vi "Cube Manipulation Logic Core v2.vi"(6 "Auto Control":bool, 8 "Manual Intake Control":dbl, 9 "Manual Lift Control":dbl, 10 "Cube Manipulation Manual Controls":T1, 11 "Cube Manipulation Button Controls":T4) -> (3 "output cluster":T2={"Control Mode"=1, "Carrage Output"=0.0, "Intake Output"=0.0, "Intake Short"=FALSE, "Intake Long"=FALSE, "Lift Output"=0.0, "Lift Output L"=0.0, "Lift Output R"=0.0} {"Control Mode" items=["PercentOutput"=0, "Position"=1, "Velocity"=2, "Current"=3, "Follower"=5, "MotionProfile"=6, "MotionMagic"=7, "MotionMagicArc"=8, "MotionProfileArc"=10, "Disabled"=15]}, 5 "Sequence Done":bool, 7 "Position Reached":bool)   [LabVIEW 2017]
uses:
  Cube Manipulation Controls.ctl
  Cube Manipulation Outputs.ctl
  <vilib>/Rock Robotics/WPI/ThirdParty/Phoenix-LabVIEW/Motor Controller/Controls/CTRE_Phoenix_MotorControl_ControlMode.ctl
  Cube Manipulation Manual Controls.ctl
  Robot Global Data.vi
panel:
  in  "Case 0 Short Hold":bool
  in  "Adjust Grip Sequence":dbl
  in  "Solinoid Buffer for Positions":dbl=5000.0 format="%#_13g"
  in  "Exchange Sequence":dbl
  in  "Buffer Zone":dbl=3500.0
  in  "Command":dbl
  in  "Sequence Position":dbl
  # "Moved Wheel \nSpeed to Global"
  # "Off= Retracted\nOn= Extended"
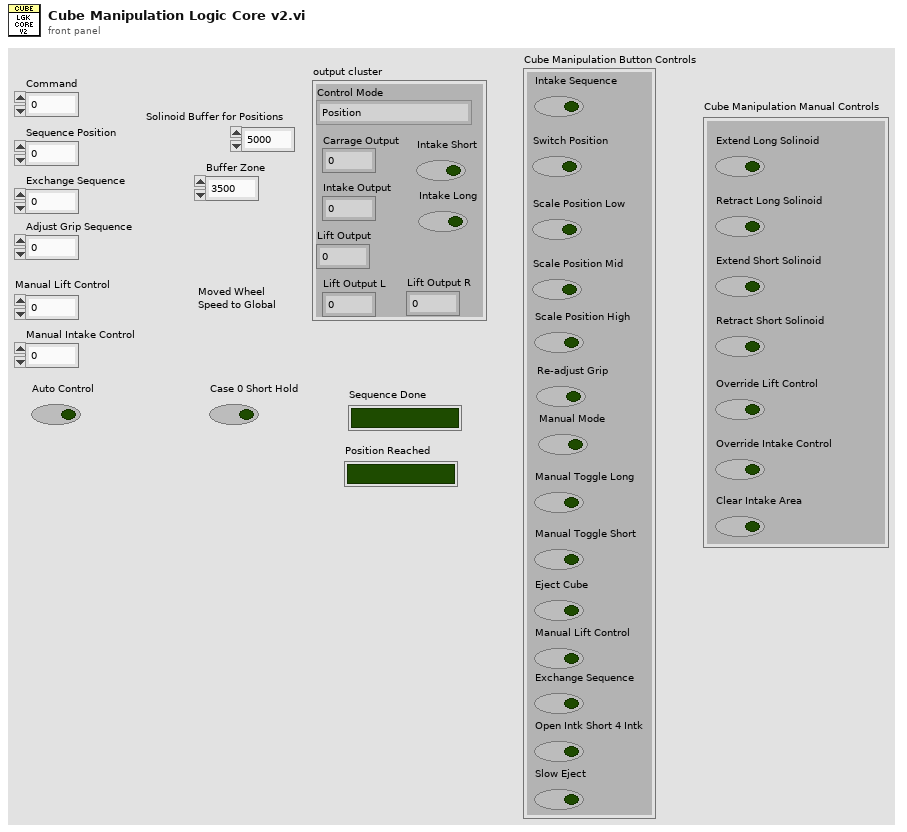
[diagram p1: front panel]
types:
  T1 = typedef "Cube Manipulation Manual Controls.ctl" = cluster{"Extend Long Solinoid":bool, "Retract Long Solinoid":bool, "Extend Short Solinoid":bool, "Retract Short Solinoid":bool, "Override Lift Control":bool, "Override Intake Control":bool, "Clear Intake Area":bool}
  T2 = typedef "Cube Manipulation Outputs.ctl" = cluster{"Control Mode":T3, "Carrage Output":dbl, "Intake Output":dbl, "Intake Short":bool, "Intake Long":bool, "Lift Output":dbl, "Lift Output L":dbl, "Lift Output R":dbl}
  T3 = typedef "CTRE_Phoenix_MotorControl_ControlMode.ctl" = u16
  T4 = typedef "Cube Manipulation Controls.ctl" = cluster{"Intake Sequence":bool, "Switch Position":bool, "Scale Position Low":bool, "Scale Position Mid":bool, "Scale Position High":bool, "Re-adjust Grip":bool, "Manual Mode":bool, "Manual Toggle Long":bool, "Manual Toggle Short":bool, "Eject Cube":bool, "Manual Lift Control":bool, "Exchange Sequence":bool, "Open Intk Short 4 Intk":bool, "Slow Eject":bool}
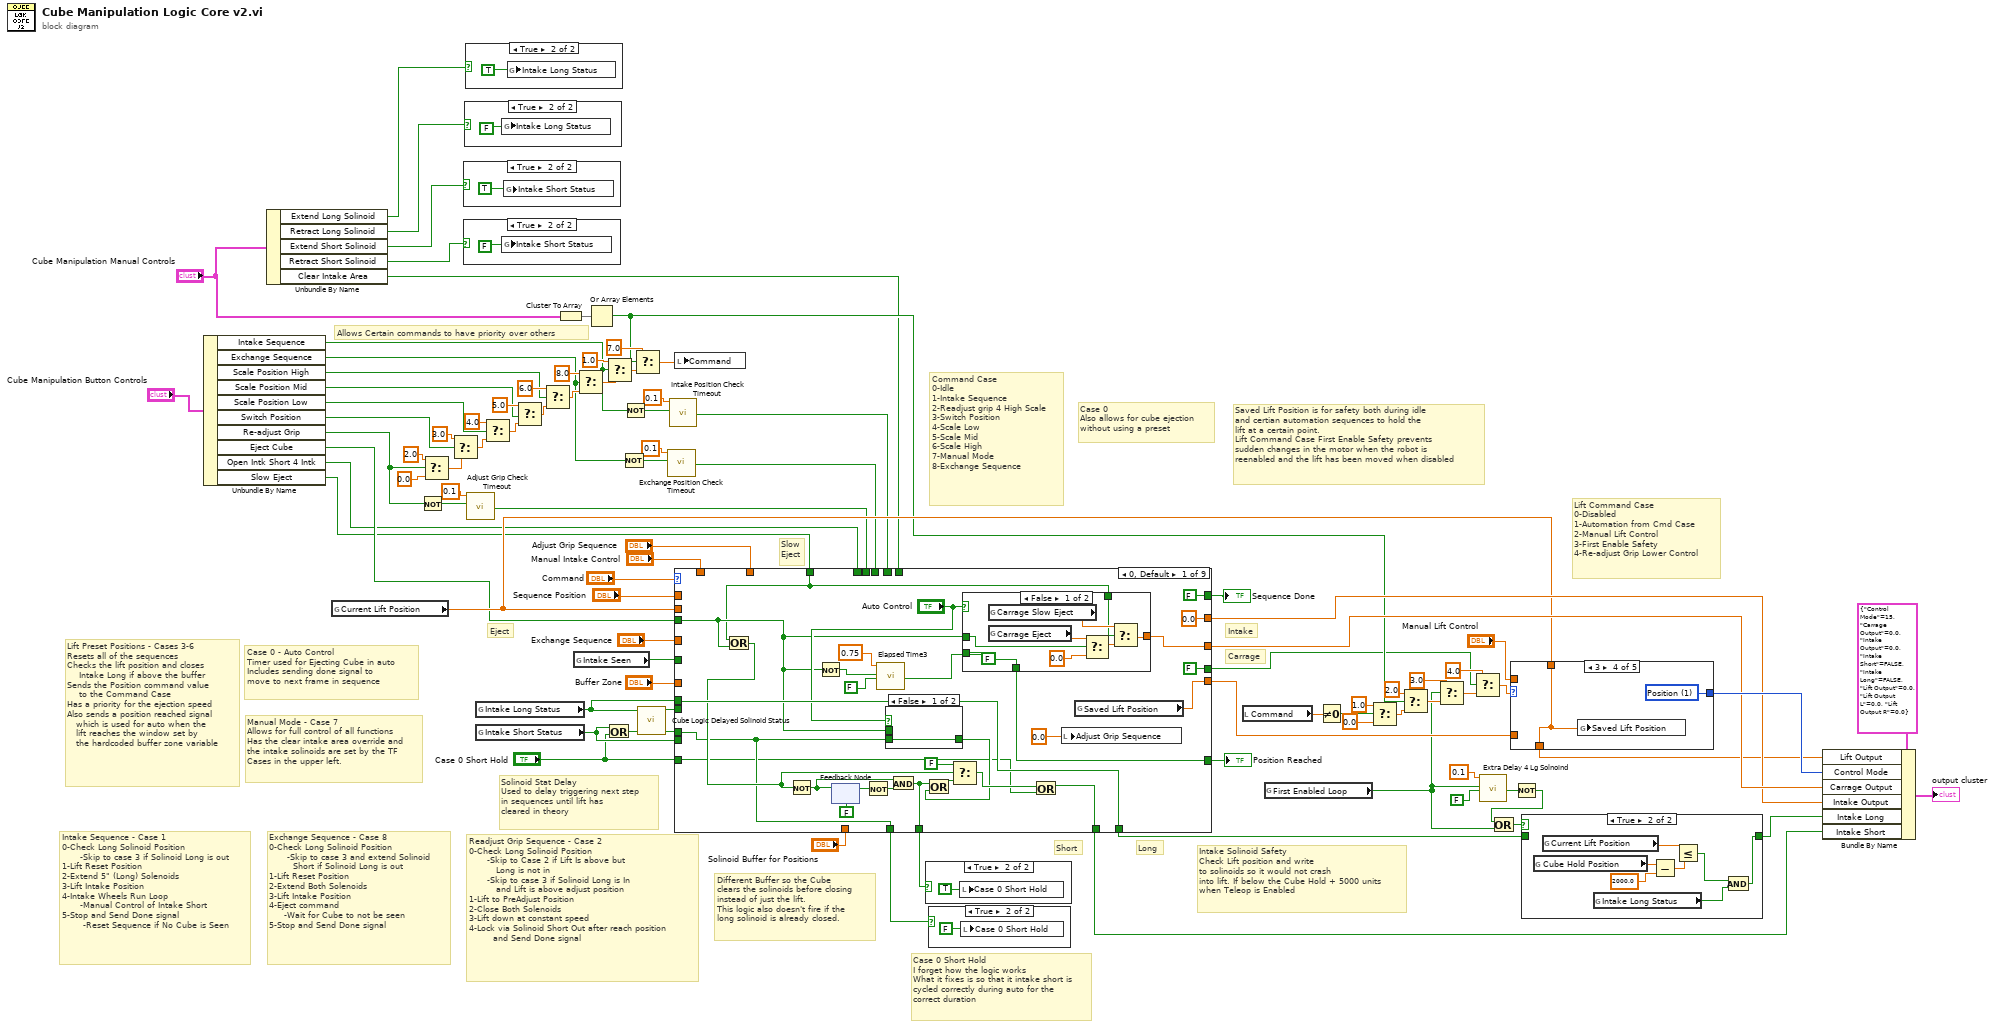
[diagram p0: block diagram]
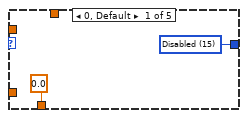
[diagram p9: hidden frame]
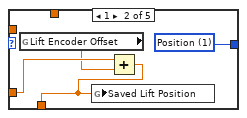
[diagram p10: hidden frame]
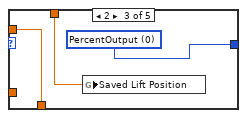
[diagram p11: hidden frame]
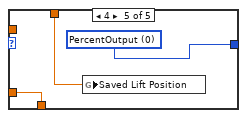
[diagram p12: hidden frame]
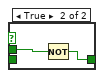
[diagram p13: hidden frame]
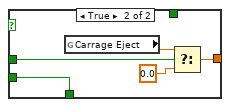
[diagram p14: hidden frame]
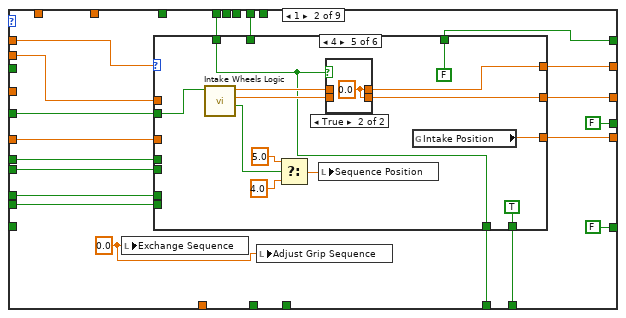
[diagram p15: hidden frame]
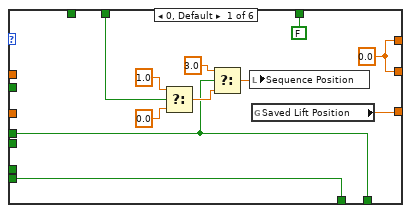
[diagram p16: hidden frame]
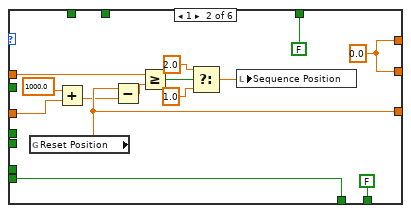
[diagram p17: hidden frame]
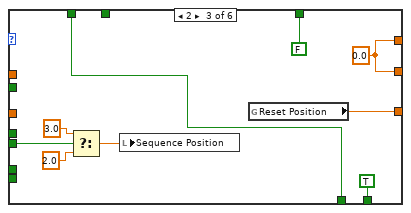
[diagram p18: hidden frame]
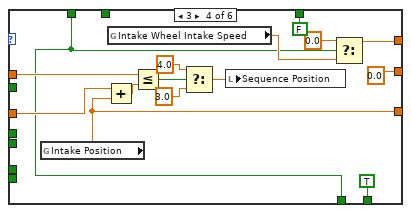
[diagram p19: hidden frame]
diagram:
  # "Allows Certain commands to have priority over others"
  # "Saved Lift Position is for safety both during idle\nand certian automation sequences to hold the\nlift at a certain point.\nLift Command Case First Enable Safety prevents\nsudden changes in the motor when the robot is \nreenabled and the lift has been moved when disabled"
  # "Case 0\nAlso allows for cube ejection\nwithout using a preset"
  # "Manual Mode - Case 7\nAllows for full control of all functions\nHas the clear intake area override and\nthe intake solinoids are set by the TF\nCases in the upper left."
  # "Lift Preset Positions - Cases 3-6\nResets all of the sequences\nChecks the lift position and closes\n    Intake Long if above the buffer\nSends the Position command value\n    to the Command Case\nHas a priority for the ejection speed\nAlso sends a position reached signal\n   which is used for auto when the \n   lift reaches the window set by\n   the hardcoded buffer zone variable"
  # "Case 0 Short Hold\nI forget how the logic works\nWhat it fixes is so that it intake short is\ncycled correctly during auto for the\ncorrect duration"
  # "Case 0 - Auto Control\nTimer used for Ejecting Cube in auto\nIncludes sending done signal to\nmove to next frame in sequence"
  # "Eject"
  # "Slow\nEject"
  # "Readjust Grip Sequence - Case 2\n0-Check Long Solinoid Position\n      -Skip to Case 2 if Lift Is above but\n         Long is not in\n      -Skip to case 3 if Solinoid Long is In\n         and Lift is above adjust position\n1-Lift to PreAdjust Position\n2-Close Both Solenoids\n3-Lift down at constant speed\n4-Lock via Solinoid Short Out after reach position\n        and Send Done signal"
  # "Carrage"
  # "Intake"
  # "Different Buffer so the Cube\nclears the solinoids before closing\ninstead of just the lift. \nThis logic also doesn't fire if the\nlong solinoid is already closed."
  # "Lift Command Case\n0-Disabled\n1-Automation from Cmd Case\n2-Manual Lift Control\n3-First Enable Safety\n4-Re-adjust Grip Lower Control"
  # "Exchange Sequence - Case 8\n0-Check Long Solinoid Position\n      -Skip to case 3 and extend Solinoid \n        Short if Solinoid Long is out\n1-Lift Reset Position\n2-Extend Both Solenoids\n3-Lift Intake Position\n4-Eject command\n     -Wait for Cube to not be seen\n5-Stop and Send Done signal"
  # "Intake Sequence - Case 1\n0-Check Long Solinoid Position\n      -Skip to case 3 if Solinoid Long is out\n1-Lift Reset Position\n2-Extend 5\" (Long) Solenoids\n3-Lift Intake Position\n4-Intake Wheels Run Loop\n      -Manual Control of Intake Short\n5-Stop and Send Done signal\n       -Reset Sequence if No Cube is Seen"
  # "Long"
  # "Short"
  # "Solinoid Stat Delay\nUsed to delay triggering next step\nin sequences until lift has \ncleared in theory"
  # "Intake Solinoid Safety\nCheck Lift position and write\nto solinoids so it would not crash\ninto lift. If below the Cube Hold + 5000 units\nwhen Teleop is Enabled"
  # "Command Case\n0-Idle\n1-Intake Sequence\n2-Readjust grip 4 High Scale\n3-Switch Position\n4-Scale Low\n5-Scale Mid\n6-Scale High\n7-Manual Mode\n8-Exchange Sequence"
  n1 = Unbundle By Name("Cube Manipulation Button Controls") -> ("Intake Sequence"=w43:bool, "Exchange Sequence"=w39:bool, "Scale Position High"=w71:bool, "Scale Position Mid"=w72:bool, "Scale Position Low"=w73:bool, "Switch Position"=w74:bool, "Re-adjust Grip"=w13:bool, "Eject Cube"=w30:bool, "Open Intk Short 4 Intk"=w21:bool, "Slow Eject"=w7:bool)
  n2 = Unbundle By Name("Cube Manipulation Manual Controls") -> ("Extend Long Solinoid"=w34:bool, "Retract Long Solinoid"=w33:bool, "Extend Short Solinoid"=w32:bool, "Retract Short Solinoid"=w31:bool, "Clear Intake Area"=w20:bool)
  n3 = global read "Robot Global Data.vi" "Current Lift Position"() -> (w64:dbl)
  n4 = Not(x=w13) -> (.not. x?=w14:bool)
  n5 = Select(t=2.0, s=w13, f=0.0) -> (s? t:f=w18:dbl)
  n6 = Select(t=3.0, s=w74, f=w18) -> (s? t:f=w91:dbl)
  n7 = case shown="True" w32 {
    frame False {
    }
    frame True {
      n8 = global write "Robot Global Data.vi" "Intake Short Status"(TRUE ("Intake Short Status")) -> ()
    }
  }
  n9 = case shown="True" w31 {
    frame False {
    }
    frame True {
      n10 = global write "Robot Global Data.vi" "Intake Short Status"(FALSE ("Intake Short Status")) -> ()
    }
  }
  n11 = case shown="True" w33 {
    frame False {
    }
    frame True {
      n12 = global write "Robot Global Data.vi" "Intake Long Status"(FALSE ("Intake Long Status")) -> ()
    }
  }
  n13 = case shown="True" w34 {
    frame False {
    }
    frame True {
      n14 = global write "Robot Global Data.vi" "Intake Long Status"(TRUE ("Intake Long Status")) -> ()
    }
  }
  n15 = call "Adjust Grip Check Timeout"("Time Target (s)"=0.1, "Reset"=w14) -> ("Time has Elapsed"=w12:bool)  [unwired: 10 in, 7 out]
  n16 = global read "Robot Global Data.vi" "Intake Long Status"() -> (w48:bool)
  n17 = global read "Robot Global Data.vi" "Intake Short Status"() -> (w4:bool)
  n18 = Select(t=4.0, s=w73, f=w91) -> (s? t:f=w92:dbl)
  n19 = Select(t=5.0, s=w72, f=w92) -> (s? t:f=w90:dbl)
  n20 = Select(t=6.0, s=w71, f=w90) -> (s? t:f=w93:dbl)
  n21 = Cluster To Array(cluster="Cube Manipulation Manual Controls") -> (array=w36:bool[])
  n22 = global read "Robot Global Data.vi" "Intake Seen"() -> (w50:bool)
  n23 = Select(t=8.0, s=w39, f=w93) -> (s? t:f=w79:dbl)
  n24 = Or Array Elements(Boolean array=w36) -> (logical OR=w23:bool)
  n25 = Or(x=w4, y="Case 0 Short Hold") -> (x .or. y?=w5:bool)
  n26 = Select(t=1.0, s=w43, f=w79) -> (s? t:f=w63:dbl)
  n27 = Not(x=w39) -> (.not. x?=w40:bool)
  n28 = Not(x=w43) -> (.not. x?=w44:bool)
  n29 = Select(t=7.0, s=w23, f=w63) -> (s? t:f=w62:dbl)
  n30 = call "Cube Logic Delayed Solinoid Status.vi"("Short Input"=w5, "Long Input"=w48) -> ("Short Delayed Output"=w56:bool, "Long Delayed Output"=w57:bool)  [unwired: 8 in]
  n31 = call "Exchange Position Check Timeout"("Time Target (s)"=0.1, "Reset"=w40) -> ("Time has Elapsed"=w38:bool)  [unwired: 10 in, 7 out]
  n32 = call "Intake Position Check Timeout"("Time Target (s)"=0.1, "Reset"=w44) -> ("Time has Elapsed"=w42:bool)  [unwired: 10 in, 7 out]
  n33 = case shown="0, Default" "Command" {
    tunnel: w64 -> [_ w160 w240 w346 w373 w398 w423 _ w480]
    tunnel: [w123 w159 w252 w349 w374 w399 w426 0.0 ("Intake Position") w479] -> w77
    tunnel: [w117 w158 w244 w339 w366 w391 w418 w453 w478] -> w49
    tunnel: [w99 w157 w245 w337 w365 w390 w417 w452 w477] -> w6
    tunnel: w57 -> [_ w156 w248 _ _ _ _ _ w476]
    tunnel: [0.0 ("Intake Output") w155 w254 0.0 ("Intake Output") 0.0 ("Intake Output") 0.0 ("Intake Output") 0.0 ("Intake Output") w455 w475] -> w67
    tunnel: [w122 w154 w253 w332 w358 w383 w410 w457 w474] -> w68
    tunnel: w56 -> [w100 w153 w247 _ _ _ _ _ w473]
    tunnel: "Sequence Position" -> [_ w152 _ _ _ _ _ _ _]
    tunnel: w30 -> [w112 _ _ w338 w357 w381 w409 w441 w469]
    tunnel: "Buffer Zone" -> [_ w151 w239 w345 w372 w395 w422 _ w472]
    tunnel: "Exchange Sequence" -> [_ _ _ _ _ _ _ _ w471]
    tunnel: [FALSE w150 w251 FALSE FALSE FALSE FALSE FALSE w470] -> w58
    tunnel: [w118 FALSE FALSE ("Time has Elapsed") w352 w375 w400 w427 FALSE FALSE] -> w55
    tunnel: w50 -> [_ w148 _ _ _ _ _ _ w466]
    tunnel: w48 -> [w117 w147 w249 w340 w367 w392 w419 w459 w467]
    tunnel: w4 -> [_ w146 w246 _ _ _ _ w435 w465]
    tunnel: w42 -> [_ w145 _ _ _ _ _ _ _]
    tunnel: w38 -> [_ _ _ _ _ _ _ _ w464]
    tunnel: "Manual Intake Control" -> [_ _ _ _ _ _ _ w443 _]
    tunnel: "Solinoid Buffer for Positions" -> [_ _ w238 w344 w371 w397 w421 _ _]
    tunnel: w21 -> [_ w144 _ _ _ _ _ _ _]
    tunnel: w20 -> [_ _ _ _ _ _ _ w450 _]
    tunnel: "Adjust Grip Sequence" -> [_ _ w250 _ _ _ _ _ _]
    tunnel: w12 -> [_ _ w242 _ _ _ _ _ _]
    tunnel: [FALSE FALSE w237 FALSE FALSE FALSE FALSE FALSE FALSE] -> w8
    tunnel: w7 -> [w111 _ _ w330 w355 w380 w407 w442 _]
    tunnel: [w101 _ _ _ _ _ _ _ _] -> w3
    tunnel: [w100 _ _ _ _ _ _ _ _] -> w2
    tunnel: "Case 0 Short Hold" -> [w98 _ _ _ _ _ _ _ _]
    frame 0, Default {
      n34 = Or(x=w111, y=w112) -> (x .or. y?=w102:bool)
      n35 = Not(x=w102) -> (.not. x?=w108:bool)
      n36 = Not(x=w112) -> (.not. x?=w115:bool)
      n37 = feedback #1(FALSE) -> (w109:bool)
      n38 = feedback-in #1(w108) -> ()
      n39 = Not(x=w109) -> (.not. x?=w110:bool)
      n40 = call "Elapsed Time3"("Time Target (s)"=0.75, "Reset"=w115, "Auto Reset"=FALSE) -> ("Time has Elapsed"=w119:bool)  [unwired: 9 in, 7 out]
      n41 = case shown="False" "Auto Control" {
        tunnel: [w126 w128] -> w103
        tunnel: w112 -> [_ w127]
        tunnel: w100 -> [w126 _]
        frame False {
        }
        frame True {
          n42 = Not(x=w127) -> (.not. x?=w128:bool)
        }
      }
      n43 = And(x=w108, y=w110) -> (x .and. y?=w101:bool)
      n44 = Or(x=w101, y=w103) -> (x .or. y?=w105:bool)
      n45 = Select(t=FALSE, s=w102, f=w105) -> (s? t:f=w104:bool)
      n46 = case shown="False" "Auto Control" {
        tunnel: [w131 w139] -> w122
        tunnel: w112 -> [w130 w138]
        tunnel: w119 -> [_ w137]
        tunnel: [FALSE w137] -> w118
        tunnel: w111 -> [w129 _]
        frame False {
          n47 = global read "Robot Global Data.vi" "Carrage Slow Eject"() -> (w133:dbl)
          n48 = global read "Robot Global Data.vi" "Carrage Eject"() -> (w134:dbl)
          n49 = Select(t=w134, s=w130, f=0.0 ("t")) -> (s? t:f=w132:dbl)
          n50 = Select(t=w133, s=w129, f=w132) -> (s? t:f=w131:dbl)
        }
        frame True {
          n51 = global read "Robot Global Data.vi" "Carrage Eject"() -> (w141:dbl)
          n52 = Select(t=w141, s=w138, f=0.0) -> (s? t:f=w139:dbl)
        }
      }
      n53 = Or(x=w104, y=w98) -> (x .or. y?=w99:bool)
      n54 = local write "Adjust Grip Sequence"(0.0 ("Exchange Sequence")) -> ()
      n55 = global read "Robot Global Data.vi" "Saved Lift Position"() -> (w123:dbl)
    }
    frame 1 {
      w143 = 0.0 ("Exchange Sequence")
      n56 = local write "Exchange Sequence"(w143) -> ()
      n57 = case shown="4" w152 {
        tunnel: w160 -> [_ w185 _ w205 _ _]
        tunnel: [w169 w178 w194 w202 w221 w236] -> w159
        tunnel: w151 -> [_ w179 _ w201 _ _]
        tunnel: [w164 FALSE TRUE TRUE TRUE TRUE] -> w158
        tunnel: [w168 w172 w186 w195 w210 FALSE ("Intake Short Status")] -> w157
        tunnel: w156 -> [_ _ w190 _ _ _]
        tunnel: [w170 w175 w187 w198 w212 w230] -> w155
        tunnel: [w170 w175 w187 0.0 ("Intake Output") w211 w230] -> w154
        tunnel: w148 -> [_ _ _ _ w216 w226]
        tunnel: w153 -> [_ _ _ _ _ _]
        tunnel: [FALSE FALSE FALSE FALSE FALSE TRUE] -> w150
        tunnel: w147 -> [w164 _ _ _ _ _]
        tunnel: w146 -> [w168 w172 _ _ _ _]
        tunnel: w145 -> [w161 _ _ _ _ _]
        tunnel: w144 -> [_ _ w186 w195 w210 _]
        frame 0, Default {
          w170 = 0.0 ("Intake Output")
          n58 = Select(t=1.0, s=w161, f=0.0) -> (s? t:f=w165:dbl)
          n59 = Select(t=3.0, s=w164, f=w165) -> (s? t:f=w166:dbl)
          n60 = local write "Sequence Position"(w166) -> ()
          n61 = global read "Robot Global Data.vi" "Saved Lift Position"() -> (w169:dbl)
        }
        frame 1 {
          w175 = 0.0 ("Intake Output")
          n62 = global read "Robot Global Data.vi" "Reset Position"() -> (w178:dbl)
          n63 = Add(x=1000.0, y=w179) -> (x+y=w174:dbl)
          n64 = Subtract(x=w178, y=w174) -> (x-y=w180:dbl)
          n65 = Greater Or Equal?(x=w185, y=w180) -> (x >= y?=w184:bool)
          n66 = Select(t=2.0, s=w184, f=1.0) -> (s? t:f=w181:dbl)
          n67 = local write "Sequence Position"(w181) -> ()
        }
        frame 2 {
          w187 = 0.0 ("Intake Output")
          n68 = Select(t=3.0, s=w190, f=2.0) -> (s? t:f=w189:dbl)
          n69 = local write "Sequence Position"(w189) -> ()
          n70 = global read "Robot Global Data.vi" "Reset Position"() -> (w194:dbl)
        }
        frame 3 {
          n71 = global read "Robot Global Data.vi" "Intake Position"() -> (w202:dbl)
          n72 = Add(x=w201, y=w202) -> (x+y=w206:dbl)
          n73 = global read "Robot Global Data.vi" "Intake Wheel Intake Speed"() -> (w197:dbl)
          n74 = Less Or Equal?(x=w205, y=w206) -> (x <= y?=w208:bool)
          n75 = Select(t=4.0, s=w208, f=3.0) -> (s? t:f=w203:dbl)
          n76 = local write "Sequence Position"(w203) -> ()
          n77 = Select(t=0.0, s=w195, f=w197) -> (s? t:f=w198:dbl)
        }
        frame 4 {
          n78 = call "Intake Wheels Logic.vi"("Intake Seen"=w216) -> ("Done"=w218:bool, "Carrage Output"=w213:dbl, "Intake Output"=w214:dbl)  [unwired: 8 in]
          n79 = Select(t=5.0, s=w218, f=4.0) -> (s? t:f=w217:dbl)
          n80 = local write "Sequence Position"(w217) -> ()
          n81 = case shown="True" w210 {
            tunnel: w214 -> [w224 _]
            tunnel: w213 -> [w223 _]
            tunnel: [w224 w225] -> w212
            tunnel: [w223 w225] -> w211
            frame False {
            }
            frame True {
              w225 = 0.0 ("Intake Output")
            }
          }
          n82 = global read "Robot Global Data.vi" "Intake Position"() -> (w221:dbl)
        }
        frame 5 {
          w230 = 0.0 ("Intake Output")
          # "Auto reset if sensors are reporting no cube detected"
          n83 = global read "Robot Global Data.vi" "Intake Secure"() -> (w228:bool)
          n84 = Not Or(1:w228, 2:w226) -> (0:w227:bool)
          n85 = Select(t=0.0, s=w227, f=5.0) -> (s? t:f=w232:dbl)
          n86 = local write "Sequence Position"(w232) -> ()
          n87 = global read "Robot Global Data.vi" "Intake Position"() -> (w236:dbl)
        }
      }
      n88 = local write "Adjust Grip Sequence"(w143) -> ()
    }
    frame 2 {
      w243 = 0.0 ("Exchange Sequence")
      n89 = local write "Exchange Sequence"(w243) -> ()
      n90 = case shown="4" w250 {
        tunnel: w240 -> [w269 w285 _ w320 _]
        tunnel: [w277 w293 0.0 ("Saved Lift Position") w313 w324] -> w252
        tunnel: w239 -> [w262 w294 _ w311 _]
        tunnel: [w274 w283 w306 w314 FALSE] -> w244
        tunnel: [w276 w280 w306 w314 FALSE ("Intake Short Status")] -> w245
        tunnel: w248 -> [_ _ w303 _ _]
        tunnel: [w278 w291 w307 w316 w324] -> w254
        tunnel: [w278 w291 w307 w316 w324] -> w253
        tunnel: [FALSE FALSE FALSE FALSE w325] -> w251
        tunnel: w249 -> [w274 w284 _ _ _]
        tunnel: w246 -> [w276 _ _ _ _]
        tunnel: w247 -> [_ _ w302 _ w325]
        tunnel: w242 -> [w271 _ _ _ _]
        tunnel: w238 -> [_ w286 _ _ _]
        tunnel: [FALSE FALSE TRUE TRUE TRUE] -> w237
        frame 0, Default {
          w278 = 0.0 ("Intake Output")
          n91 = global read "Robot Global Data.vi" "PreAdjust Position"() -> (w268:dbl)
          n92 = Add(x=1000.0, y=w262) -> (x+y=w261:dbl)
          n93 = Subtract(x=w268, y=w261) -> (x-y=w270:dbl)
          n94 = Greater Or Equal?(x=w269, y=w270) -> (x >= y?=w264:bool)
          n95 = Select(t=1.0, s=w271, f=0.0) -> (s? t:f=w259:dbl)
          n96 = Not(x=w264) -> (.not. x?=w265:bool)
          n97 = call "Adjust Grip Check Timeout2"("Time Target (s)"=0.05, "Reset"=w265) -> ("Time has Elapsed"=w266:bool)  [unwired: 10 in, 7 out]
          n98 = And(x=w264, y=w274) -> (x .and. y?=w256:bool)
          n99 = Select(t=2.0, s=w266, f=w259) -> (s? t:f=w257:dbl)
          n100 = global read "Robot Global Data.vi" "Saved Lift Position"() -> (w277:dbl)
          n101 = Select(t=3.0, s=w256, f=w257) -> (s? t:f=w275:dbl)
          n102 = local write "Adjust Grip Sequence"(w275) -> ()
        }
        frame 1 {
          w291 = 0.0 ("Intake Output")
          n103 = global read "Robot Global Data.vi" "PreAdjust Position"() -> (w293:dbl)
          n104 = Add(x=1000.0, y=w294) -> (x+y=w290:dbl)
          n105 = global read "Robot Global Data.vi" "Cube Hold Position"() -> (w288:dbl)
          n106 = Subtract(x=w293, y=w290) -> (x-y=w295:dbl)
          n107 = Greater Or Equal?(x=w285, y=w295) -> (x >= y?=w299:bool)
          n108 = Select(t=2.0, s=w299, f=1.0) -> (s? t:f=w296:dbl)
          n109 = Add(x=w288, y=w286) -> (x+y=w287:dbl)
          n110 = local write "Adjust Grip Sequence"(w296) -> ()
          n111 = Less Or Equal?(x=w285, y=w287) -> (x <= y?=w281:bool)
          n112 = Not(x=w281) -> (.not. x?=w280:bool)
          n113 = And(x=w284, y=w281) -> (x .and. y?=w283:bool)
        }
        frame 2 {
          w307 = 0.0 ("Intake Output")
          w306 = FALSE
          n114 = Not Or(1:w302, 2:w303) -> (0:w304:bool)
          n115 = Select(t=3.0, s=w304, f=2.0) -> (s? t:f=w305:dbl)
          n116 = local write "Adjust Grip Sequence"(w305) -> ()
        }
        frame 3 {
          w314 = FALSE ("Intake Short Status")
          w316 = 0.0 ("Intake Output")
          n117 = global read "Robot Global Data.vi" "Adjusted Position"() -> (w318:dbl)
          n118 = Add(x=w311, y=w318) -> (x+y=w321:dbl)
          n119 = Less Or Equal?(x=w320, y=w321) -> (x <= y?=w323:bool)
          n120 = Select(t=4.0, s=w323, f=3.0) -> (s? t:f=w315:dbl)
          n121 = global read "Robot Global Data.vi" "Adjust Position Speed"() -> (w313:dbl)
          n122 = local write "Adjust Grip Sequence"(w315) -> ()
        }
        frame 4 {
          w324 = 0.0 ("Intake Output")
          n123 = local write "Adjust Grip Sequence"(4.0 ("Adjust Grip Sequence")) -> ()
        }
      }
      n124 = local write "Sequence Position"(w243) -> ()
    }
    frame 3 {
      w336 = 0.0 ("Sequence Position")
      n125 = local write "Sequence Position"(w336) -> ()
      n126 = local write "Exchange Sequence"(w336) -> ()
      n127 = local write "Adjust Grip Sequence"(w336) -> ()
      n128 = global read "Robot Global Data.vi" "Cube Hold Position"() -> (w343:dbl)
      n129 = Add(x=w343, y=w344) -> (x+y=w342:dbl)
      n130 = Less Or Equal?(x=w346, y=w342) -> (x <= y?=w341:bool)
      n131 = And(x=w340, y=w341) -> (x .and. y?=w339:bool)
      n132 = global read "Robot Global Data.vi" "Carrage Slow Eject"() -> (w334:dbl)
      n133 = global read "Robot Global Data.vi" "Carrage Eject"() -> (w347:dbl)
      n134 = Or(x=w338, y=w330) -> (x .or. y?=w331:bool)
      n135 = global read "Robot Global Data.vi" "Switch Position"() -> (w349:dbl)
      n136 = Not(x=w331) -> (.not. x?=w337:bool)
      n137 = Select(t=w347, s=w338, f=0.0 ("t")) -> (s? t:f=w333:dbl)
      n138 = Add(x=w349, y=w345) -> (x+y=w351:dbl)
      n139 = Subtract(x=w349, y=w345) -> (x-y=w350:dbl)
      n140 = Select(t=w334, s=w330, f=w333) -> (s? t:f=w332:dbl)
      n141 = In Range and Coerce(upper limit=w351, x=w346, lower limit=w350) -> (In Range?=w352:bool)  [unwired: 1 out]
    }
    frame 4 {
      w364 = 0.0 ("Sequence Position")
      n142 = global read "Robot Global Data.vi" "Cube Hold Position"() -> (w370:dbl)
      n143 = local write "Adjust Grip Sequence"(w364) -> ()
      n144 = local write "Sequence Position"(w364) -> ()
      n145 = local write "Exchange Sequence"(w364) -> ()
      n146 = Add(x=w370, y=w371) -> (x+y=w369:dbl)
      n147 = Less Or Equal?(x=w373, y=w369) -> (x <= y?=w368:bool)
      n148 = And(x=w367, y=w368) -> (x .and. y?=w366:bool)
      n149 = global read "Robot Global Data.vi" "Scale Position Low"() -> (w374:dbl)
      n150 = global read "Robot Global Data.vi" "Carrage Slow Eject"() -> (w360:dbl)
      n151 = global read "Robot Global Data.vi" "Carrage Eject"() -> (w361:dbl)
      n152 = Or(x=w357, y=w355) -> (x .or. y?=w356:bool)
      n153 = Not(x=w356) -> (.not. x?=w365:bool)
      n154 = Select(t=w361, s=w357, f=0.0 ("t")) -> (s? t:f=w359:dbl)
      n155 = Add(x=w374, y=w372) -> (x+y=w377:dbl)
      n156 = Subtract(x=w374, y=w372) -> (x-y=w376:dbl)
      n157 = Select(t=w360, s=w355, f=w359) -> (s? t:f=w358:dbl)
      n158 = In Range and Coerce(upper limit=w377, x=w373, lower limit=w376) -> (In Range?=w375:bool)  [unwired: 1 out]
    }
    frame 5 {
      w389 = 0.0 ("Sequence Position")
      n159 = local write "Adjust Grip Sequence"(w389) -> ()
      n160 = local write "Sequence Position"(w389) -> ()
      n161 = local write "Exchange Sequence"(w389) -> ()
      n162 = global read "Robot Global Data.vi" "Cube Hold Position"() -> (w396:dbl)
      n163 = Add(x=w396, y=w397) -> (x+y=w394:dbl)
      n164 = Less Or Equal?(x=w398, y=w394) -> (x <= y?=w393:bool)
      n165 = And(x=w392, y=w393) -> (x .and. y?=w391:bool)
      n166 = global read "Robot Global Data.vi" "Scale Position Mid"() -> (w399:dbl)
      n167 = global read "Robot Global Data.vi" "Carrage Slow Eject"() -> (w385:dbl)
      n168 = global read "Robot Global Data.vi" "Carrage Eject"() -> (w386:dbl)
      n169 = Or(x=w381, y=w380) -> (x .or. y?=w382:bool)
      n170 = Not(x=w382) -> (.not. x?=w390:bool)
      n171 = Select(t=w386, s=w381, f=0.0 ("t")) -> (s? t:f=w384:dbl)
      n172 = Add(x=w399, y=w395) -> (x+y=w402:dbl)
      n173 = Subtract(x=w399, y=w395) -> (x-y=w401:dbl)
      n174 = Select(t=w385, s=w380, f=w384) -> (s? t:f=w383:dbl)
      n175 = In Range and Coerce(upper limit=w402, x=w398, lower limit=w401) -> (In Range?=w400:bool)  [unwired: 1 out]
    }
    frame 6 {
      w416 = 0.0 ("Sequence Position")
      n176 = local write "Exchange Sequence"(w416) -> ()
      n177 = local write "Sequence Position"(w416) -> ()
      n178 = local write "Adjust Grip Sequence"(w416) -> ()
      n179 = global read "Robot Global Data.vi" "Cube Hold Position"() -> (w424:dbl)
      n180 = Add(x=w424, y=w421) -> (x+y=w425:dbl)
      n181 = Less Or Equal?(x=w423, y=w425) -> (x <= y?=w420:bool)
      n182 = And(x=w419, y=w420) -> (x .and. y?=w418:bool)
      n183 = global read "Robot Global Data.vi" "Scale Position High"() -> (w426:dbl)
      n184 = Or(x=w409, y=w407) -> (x .or. y?=w408:bool)
      n185 = global read "Robot Global Data.vi" "Carrage Slow Eject"() -> (w412:dbl)
      n186 = global read "Robot Global Data.vi" "Carrage Eject"() -> (w413:dbl)
      n187 = Not(x=w408) -> (.not. x?=w417:bool)
      n188 = Add(x=1500.0, y=w422) -> (x+y=w406:dbl)
      n189 = Select(t=w413, s=w409, f=0.0 ("t")) -> (s? t:f=w411:dbl)
      n190 = Select(t=w412, s=w407, f=w411) -> (s? t:f=w410:dbl)
      n191 = Subtract(x=w426, y=w406) -> (x-y=w428:dbl)
      n192 = Greater Or Equal?(x=w423, y=w428) -> (x >= y?=w427:bool)
    }
    frame 7 {
      w449 = 0.0 ("Sequence Position")
      # "Controls\nFwd=Eject\nBkwd=Intake"
      # "Carrage\nEject=Postive\nIn=Neg"
      # "Intake\nEject=Neg\nIn=Positive"
      # "Controller\nFwd=Negative\nBkwd=Positive"
      n193 = global read "Robot Global Data.vi" "Carrage Slow Eject"() -> (w446:dbl)
      n194 = global read "Robot Global Data.vi" "Carrage Eject"() -> (w447:dbl)
      n195 = Or(x=w442, y=w441) -> (x .or. y?=w433:bool)
      n196 = Not(x=w433) -> (.not. x?=w438:bool)
      n197 = feedback #2(FALSE) -> (w439:bool)
      n198 = feedback-in #2(w438) -> ()
      n199 = Not(x=w439) -> (.not. x?=w440:bool)
      n200 = And(x=w438, y=w440) -> (x .and. y?=w436:bool)
      n201 = Select(t=w447, s=w441, f=w443) -> (s? t:f=w445:dbl)
      n202 = Less Than 0?(x=w443) -> (x < 0?=w431:bool)
      n203 = Or(x=w435, y=w436) -> (x .or. y?=w434:bool)
      n204 = Select(t=w446, s=w442, f=w445) -> (s? t:f=w444:dbl)
      n205 = Or(x=w431, y=w433) -> (x .or. y?=w432:bool)
      n206 = Select(t=FALSE ("Intake Short Status"), s=w432, f=w434) -> (s? t:f=w451:bool)
      n207 = local write "Adjust Grip Sequence"(w449) -> ()
      n208 = local write "Sequence Position"(w449) -> ()
      n209 = local write "Exchange Sequence"(w449) -> ()
      n210 = Or(x=w450, y=w459) -> (x .or. y?=w453:bool)
      n211 = Or(x=w450, y=w451) -> (x .or. y?=w452:bool)
      n212 = Select(t=-1.0, s=w450, f=w444) -> (s? t:f=w455:dbl)
      n213 = Negate(x=w455) -> (-x=w457:dbl)
    }
    frame 8 {
      w463 = 0.0 ("Sequence Position")
      n214 = local write "Sequence Position"(w463) -> ()
      n215 = case shown="3" w471 {
        tunnel: w480 -> [_ w505 _ w523 _ _]
        tunnel: [w491 w498 w515 w520 w539 w547] -> w479
        tunnel: w472 -> [_ w499 _ w519 _ _]
        tunnel: [w482 w494 w514 w518 TRUE TRUE] -> w478
        tunnel: [w483 w495 w514 w518 FALSE FALSE ("Intake Short Status")] -> w477
        tunnel: w476 -> [_ _ w508 _ _ _]
        tunnel: [w489 w496 w506 w516 w534 w546] -> w475
        tunnel: [w489 w496 w506 w516 w535 w546] -> w474
        tunnel: w473 -> [_ _ w510 _ _ _]
        tunnel: [FALSE FALSE FALSE FALSE FALSE TRUE] -> w470
        tunnel: w466 -> [_ _ _ _ w536 _]
        tunnel: w469 -> [_ _ _ _ w531 _]
        tunnel: w467 -> [w482 w494 _ _ _ _]
        tunnel: w465 -> [w484 w495 _ _ _ _]
        tunnel: w464 -> [w487 _ _ _ _ _]
        frame 0, Default {
          w489 = 0.0 ("Intake Output")
          n216 = Select(t=1.0, s=w487, f=0.0) -> (s? t:f=w488:dbl)
          n217 = Select(t=3.0, s=w482, f=w488) -> (s? t:f=w492:dbl)
          n218 = local write "Exchange Sequence"(w492) -> ()
          n219 = global read "Robot Global Data.vi" "Saved Lift Position"() -> (w491:dbl)
          n220 = Select(t=TRUE, s=w482, f=w484) -> (s? t:f=w483:bool)
        }
        frame 1 {
          w496 = 0.0 ("Intake Output")
          n221 = global read "Robot Global Data.vi" "Reset Position"() -> (w498:dbl)
          n222 = Subtract(x=w498, y=w499) -> (x-y=w500:dbl)
          n223 = Greater Or Equal?(x=w505, y=w500) -> (x >= y?=w504:bool)
          n224 = Select(t=2.0, s=w504, f=1.0) -> (s? t:f=w501:dbl)
          n225 = local write "Exchange Sequence"(w501) -> ()
        }
        frame 2 {
          w514 = TRUE
          w506 = 0.0 ("Intake Output")
          n226 = And(x=w508, y=w510) -> (x .and. y?=w509:bool)
          n227 = Select(t=3.0, s=w509, f=2.0) -> (s? t:f=w511:dbl)
          n228 = local write "Exchange Sequence"(w511) -> ()
          n229 = global read "Robot Global Data.vi" "Reset Position"() -> (w515:dbl)
        }
        frame 3 {
          w516 = 0.0 ("Intake Output")
          w518 = TRUE
          n230 = global read "Robot Global Data.vi" "Intake Position"() -> (w520:dbl)
          n231 = Add(x=w519, y=w520) -> (x+y=w524:dbl)
          n232 = Less Or Equal?(x=w523, y=w524) -> (x <= y?=w526:bool)
          n233 = Select(t=4.0, s=w526, f=3.0) -> (s? t:f=w521:dbl)
          n234 = local write "Exchange Sequence"(w521) -> ()
        }
        frame 4 {
          n235 = Not(x=w536) -> (.not. x?=w530:bool)
          n236 = Select(t=5.0, s=w530, f=4.0) -> (s? t:f=w540:dbl)
          n237 = global read "Robot Global Data.vi" "Carrage Eject"() -> (w529:dbl)
          n238 = local write "Exchange Sequence"(w540) -> ()
          n239 = global read "Robot Global Data.vi" "Intake Position"() -> (w539:dbl)
          n240 = Select(t=w529, s=w531, f=0.0) -> (s? t:f=w535:dbl)
          n241 = Select(t=-1.0 ("Intake Output"), s=w531, f=0.0) -> (s? t:f=w534:dbl)
        }
        frame 5 {
          w546 = 0.0 ("Intake Output")
          n242 = local write "Exchange Sequence"(5.0 ("Exchange Sequence")) -> ()
          n243 = global read "Robot Global Data.vi" "Intake Position"() -> (w547:dbl)
        }
      }
      n244 = local write "Adjust Grip Sequence"(w463) -> ()
    }
  }
  "Sequence Done" <- w58
  "Position Reached" <- w55
  n245 = local write "Command"(w62) -> ()
  n246 = case shown="True" w3 {
    frame False {
    }
    frame True {
      n247 = local write "Case 0 Short Hold"(TRUE ("Case 0 Short Hold")) -> ()
    }
  }
  n248 = case shown="True" w2 {
    frame False {
    }
    frame True {
      n249 = local write "Case 0 Short Hold"(FALSE ("Case 0 Short Hold")) -> ()
    }
  }
  n250 = local read "Command"() -> (w52:dbl)
  n251 = global read "Robot Global Data.vi" "First Enabled Loop"() -> (w27:bool)
  n252 = Not Equal To 0?(x=w52) -> (x != 0?=w82:bool)
  n253 = Select(t=1.0, s=w82, f=0.0) -> (s? t:f=w84:dbl)
  n254 = Select(t=2.0, s=w23, f=w84) -> (s? t:f=w54:dbl)
  n255 = Select(t=3.0, s=w27, f=w54) -> (s? t:f=w10:dbl)
  n256 = Select(t=4.0, s=w8, f=w10) -> (s? t:f=w11:dbl)
  n257 = call "Extra Delay 4 Lg Solnoind"("Time Target (s)"=0.1, "Reset"=w27, "Auto Reset"=FALSE) -> ("Time has Elapsed"=w26:bool)  [unwired: 9 in, 7 out]
  n258 = case shown="3" w11 {
    tunnel: "Manual Lift Control" -> [_ _ w558 _ _]
    tunnel: w77 -> [_ w554 _ _ w562]
    tunnel: w64 -> [_ _ w557 w560 w563]
    tunnel: [w552 w556 w559 w561 w564] -> w69
    tunnel: [0.0 ("Current Lift Position") w555 w558 w560 w562] -> w65
    frame 0, Default {
      w552 = T3 15 items=["PercentOutput"=0, "Position"=1, "Velocity"=2, "Current"=3, "Follower"=5, "MotionProfile"=6, "MotionMagic"=7, "MotionMagicArc"=8, "MotionProfileArc"=10, "Disabled"=15] ("Control Mode")
    }
    frame 1 {
      w556 = T3 1 items=["PercentOutput"=0, "Position"=1, "Velocity"=2, "Current"=3, "Follower"=5, "MotionProfile"=6, "MotionMagic"=7, "MotionMagicArc"=8, "MotionProfileArc"=10, "Disabled"=15] ("Control Mode")
      n259 = global read "Robot Global Data.vi" "Lift Encoder Offset"() -> (w553:dbl)
      n260 = Add(x=w554, y=w553) -> (x+y=w555:dbl)
      n261 = global write "Robot Global Data.vi" "Saved Lift Position"(w555) -> ()
    }
    frame 2 {
      w559 = T3 0 items=["PercentOutput"=0, "Position"=1, "Velocity"=2, "Current"=3, "Follower"=5, "MotionProfile"=6, "MotionMagic"=7, "MotionMagicArc"=8, "MotionProfileArc"=10, "Disabled"=15] ("Control Mode")
      n262 = global write "Robot Global Data.vi" "Saved Lift Position"(w557) -> ()
    }
    frame 3 {
      w561 = T3 1 items=["PercentOutput"=0, "Position"=1, "Velocity"=2, "Current"=3, "Follower"=5, "MotionProfile"=6, "MotionMagic"=7, "MotionMagicArc"=8, "MotionProfileArc"=10, "Disabled"=15] ("Control Mode")
      n263 = global write "Robot Global Data.vi" "Saved Lift Position"(w560) -> ()
    }
    frame 4 {
      w564 = T3 0 items=["PercentOutput"=0, "Position"=1, "Velocity"=2, "Current"=3, "Follower"=5, "MotionProfile"=6, "MotionMagic"=7, "MotionMagicArc"=8, "MotionProfileArc"=10, "Disabled"=15] ("Control Mode")
      n264 = global write "Robot Global Data.vi" "Saved Lift Position"(w563) -> ()
    }
  }
  n265 = Not(x=w26) -> (.not. x?=w24:bool)
  n266 = Or(x=w24, y=w27) -> (x .or. y?=w25:bool)
  n267 = case shown="True" w25 {
    tunnel: [w565 w567] -> w47
    tunnel: w49 -> [w565 _]
    frame False {
    }
    frame True {
      n268 = global read "Robot Global Data.vi" "Cube Hold Position"() -> (w572:dbl)
      n269 = global read "Robot Global Data.vi" "Current Lift Position"() -> (w570:dbl)
      n270 = global read "Robot Global Data.vi" "Intake Long Status"() -> (w568:bool)
      n271 = Subtract(x=w572, y=2000.0) -> (x-y=w571:dbl)
      n272 = Less Or Equal?(x=w570, y=w571) -> (x <= y?=w566:bool)
      n273 = And(x=w566, y=w568) -> (x .and. y?=w567:bool)
    }
  }
  n274 = Bundle By Name(cluster=T2 {"Control Mode"=15, "Carrage Output"=0.0, "Intake Output"=0.0, "Intake Short"=FALSE, "Intake Long"=FALSE, "Lift Output"=0.0, "Lift Output L"=0.0, "Lift Output R"=0.0}, "Lift Output"=w65, "Control Mode"=w69, "Carrage Output"=w68, "Intake Output"=w67, "Intake Long"=w47, "Intake Short"=w6) -> (→"output cluster":T2)
